vi "resetPreconditioningCycles.vi"(8 "error in (no error)":errorcluster, 11 "Model in":refnum<class "Model.lvclass">) -> (0 "error out":errorcluster, 3 "Model out":refnum<class "Model.lvclass">)   [LabVIEW 2015, in "Model.lvclass"]
uses:
  Model.lvclass
  Model.lvclass/Model.ctl
  ApplicationElements/PreconditioningMonitor/PreconditioningMonitor.lvclass
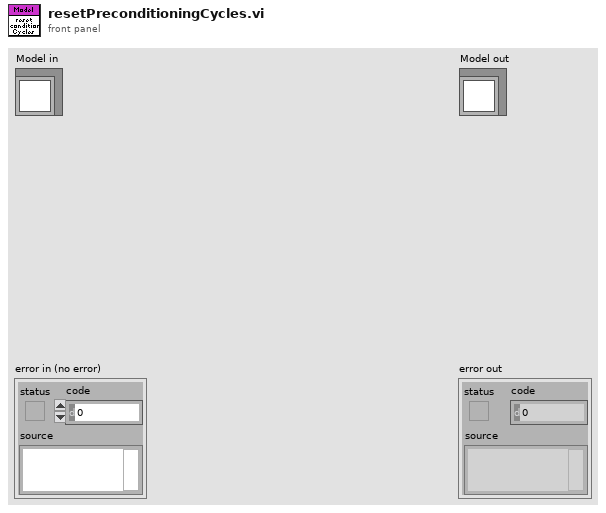
[diagram p1: front panel]
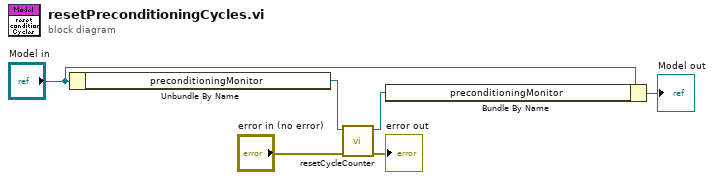
[diagram p0: block diagram]
diagram:
  n1 = Unbundle By Name("Model in") -> ("preconditioningMonitor"=w6:refnum<class "PreconditioningMonitor.lvclass">)
  n2 = call "resetCycleCounter.vi"("error in (no error)"="error in (no error)", "PreconditioningMonitor in"=w6) -> ("error out"=→"error out":errorcluster, "PreconditioningMonitor out"=w5:refnum<class "PreconditioningMonitor.lvclass">)  [unwired: 8 in]
  n3 = Bundle By Name(cluster="Model in", "preconditioningMonitor"=w5) -> (→"Model out":refnum<class "Model.lvclass">)
